vi "inverseKinematicssubVi.vi"(10 "y":dbl, 11 "x":dbl) -> (2 "second joint":dbl, 3 "first joint":dbl)   [LabVIEW 2014]
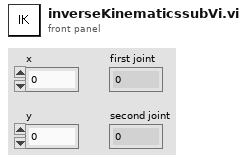
[diagram p1: front panel]
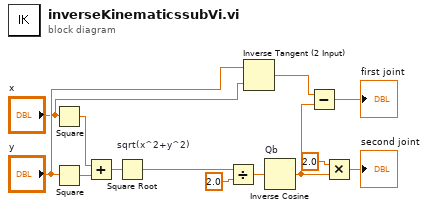
[diagram p0: block diagram]
diagram:
  n1 = Square(x="x") -> (x^2=w5:dbl)
  n2 = Square(x="y") -> (x^2=w4:dbl)
  n3 = Add(x=w5, y=w4) -> (x+y=w6:dbl)
  n4 = Square Root "sqrt(x^2+y^2)"(x=w6) -> (sqrt(x)=w7:dbl)
  n5 = Divide(x=w7, y=2.0) -> (x/y=w9:dbl)
  n6 = Inverse Tangent (2 Input)(1:"x", 2:"y") -> (0:w1:dbl)
  n7 = Inverse Cosine "Qb"(1:w9) -> (0:w13:dbl)
  n8 = Subtract(x=w1, y=w13) -> (x-y=→"first joint":dbl)
  n9 = Multiply(x=2.0, y=w13) -> (x*y=→"second joint":dbl)
